vi "HatchPosition.vi"(9 "Boolean":bool, 10 "Bitmap":u32[][](array[colorbox]), 11 "Refnum in":T1) -> (3 "Refnum out":T1)   [LabVIEW 2018]
uses:
  <vilib>/vision/Image Controls.llb/IMAQ Image.ctl
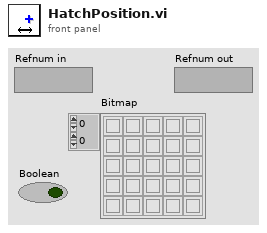
[diagram p1: front panel]
types:
  T1 = typedef "IMAQ Image.ctl" = refnum<image>
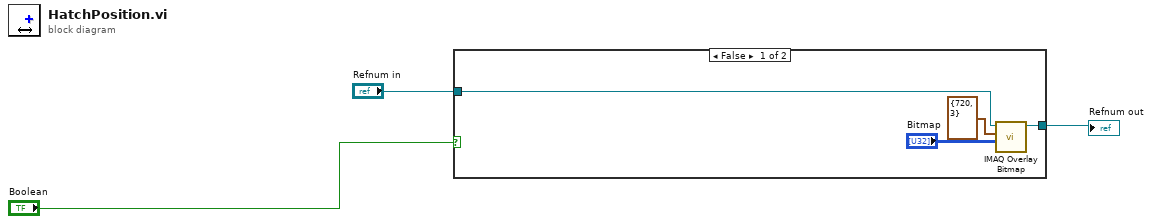
[diagram p0: block diagram]
diagram:
  n1 = case shown="False" "Boolean" {
    tunnel: "Refnum in" -> [w6 w8]
    tunnel: [w7 w8] -> w2
    frame False {
      n2 = call "IMAQ Overlay Bitmap"("Bitmap"="Bitmap", "Top Left Point"=cluster{"X":i32, "Y":i32} {"X"=720, "Y"=3}, "Image"=w6) -> ("Image Out"=w7:T1)  [unwired: 7 in, 1 out]
    }
    frame True {
    }
  }
  "Refnum out" <- w2
